vi "Sent file reference to queue.vi"(8 "error in (no error)":errorcluster, 9 "Send?":bool, 10 "Queue in":refnum<queue>, 11 "Write Region Reference":refnum<data-value>) -> (0 "error out":errorcluster, 3 "Data Value Reference out":refnum<data-value>)   [LabVIEW 2018]
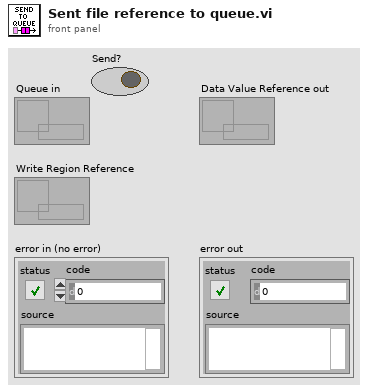
[diagram p1: front panel]
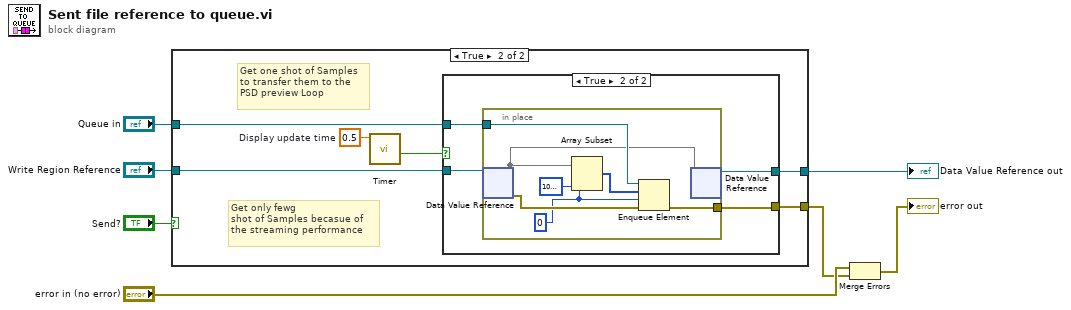
[diagram p0: block diagram]
diagram:
  n1 = case shown="True" "Send?" {
    tunnel: "Write Region Reference" -> [w8 w11]
    tunnel: "Queue in" -> [_ w12]
    tunnel: [_ w14] -> w5
    tunnel: [w8 w10] -> w4
    frame False {
    }
    frame True {
      w13 = 0.5  # Display update time
      # "Get only fewg\nshot of Samples becasue of \nthe streaming performance"
      # "Get one shot of Samples\nto transfer them to the \nPSD preview Loop"
      n2 = call "Timer.vi"("Set Time [s]"=w13) -> ("Time elapsed!"=w9:bool)  [unwired: 9 in, 1 out]
      n3 = case shown="True" w9 {
        tunnel: w12 -> [_ w19]
        tunnel: w11 -> [w15 w16]
        tunnel: [w15 w18] -> w10
        tunnel: [_ w17] -> w14
        frame False {
        }
        frame True {
          n4 = in-place {
            in-place-border: w19 -> [w26]
            in-place-border: [w24] -> w17
            w20 = 0 ("timeout in ms (-1)")
            n5 = in-place-dvr #1(w16) -> (w23:u64[], w25:errorcluster)
            n6 = Array Subset(array=w23, index=w20, length=1000000 ("index")) -> (w22:u64[])
            n7 = Enqueue Element(queue=w26, element=w22, timeout in ms (-1)=w20, error in (no error)=w25) -> (error out=w24:errorcluster)  [unwired: 2 out]
            n8 = in-place-dvr #1(w23) -> (w18:refnum<data-value>)  [unwired: 1 out]
          }
        }
      }
    }
  }
  "Data Value Reference out" <- w4
  n9 = Merge Errors("error in (no error)", w5) -> (→"error out":errorcluster)
